vi "AODScanner_6_May_2014.vi"() -> ()   [LabVIEW 2012]
uses:
  AODAcq/AODAcq.lvclass
  <vilib>/rvi/interface/nirviReadWriteControl/nirviReadWriteControl.xnode
  FPGA_Control/AODRef.ctl
  <vilib>/rvi/interface/nirviMethod/nirviMethod.xnode
  <vilib>/rvi/errors/niLvFpgaMergeErrorWithErrorCode.vi
  Motion Stabilization/GlobalVars.vi
  <vilib>/DAQmx/write.llb/DAQmx Write (Analog DBL 1Chan 1Samp).vi
  <vilib>/DAQmx/read.llb/DAQmx Read (Analog Wfm 1Chan NSamp).vi
panel:
  out "Motion FIFO":refnum<queue>
  out "Motion ROIs":T1(array[cluster])
  out "Motion Plane Centers":i32[][](array[numeric])
  out "Number of Motion Planes":i32
  in  "Motion rate (Hz) 2":dbl=10.0
  out "error out 3":errorcluster
  out "Out Points":i32[][](array[numeric])
  out "Y-Z Motion Points":i32[][](array[numeric])
  out "X-Y Motion Points":i32[][](array[numeric])
  out "Points_um":dbl[][](array[numeric])
  out "Lens Magnification":i32=20
  in  "Matlab Server Shared Folder":string="c:\\temp"
  in  "Matlab Server IP Address":string="10.21.16.18"
  in  "External Magnification":dbl=1.3
  out "error out 2":errorcluster
  out "Objective Position":cluster{"X":dbl, "Y":dbl, "Z":dbl}
  out "Numeric":i32=299
  out "error out":errorcluster
  out "ROIs":T1(array[cluster])
  out "Histogram":dynamicdata(graph)
  out "Raw samples remaining":u32
  out "Temporal samples remaining":u32
  out "Motion samples remaining":u32
  out "Image samples remaining":u32
  out "Recording File":path
  out "Waveform Chart":waveform(dbl)(graph)
  out "Ephys":bool
  in  "TraceElements":u32=10000
  out "ScanProgress":dbl(slide) scale=0.0..1.0
  in  "Abort":bool
  out "Progress":dbl(slide) scale=0.0..1.0
  in  "SweepSettings":bool
  in  "stop":bool
  in  "Power":dbl(slide)=2.5 min=0.0 max=5.0 step=0.1 scale=0.0..2.5
  out "Scan":bool
  out "Volume":bool
  in  "Tab Control":enum32{"Setup", "Volume", "Traces", "Motion"}(tab)
  in  "Store Raw":bool
  in  "Disp Volume":bool=TRUE
  in  "Save Volume":bool
  in  "Ephys":bool
  in  "Motion rate (Hz)":dbl=10.0
  in  "Scan Settings (um)":T2={"XStart"=-100, "XEnd"=100, "XNum"=250, "YStart"=-100, "YEnd"=100, "YNum"=250, "ZStart"=-30, "ZEnd"=70, "ZNum"=60}
  in  "Objective":enum16{"20x Olympus"}(ring)
  in  "Scan Time (s)":dbl=300.0
  in  "Volume Reps":i32=1 min=1 max=10000
  in  "Volume":bool
  in  "Scan":bool
  in  "Motion Channel To Analyze":i32=2 min=1 max=2
  in  "Motion Analysis":bool
  in  "Per Cell Motion Analysis":bool
  in  "Sampling Structure":u16(ring) items=["Cube Vertices"]
  in  "Auto Motion Plane Params":T3={"XY Offset"=3, "Z Offset"=6, "Line Length"=12.0, "Box Size"=12.0, "Number of Planes Per Point"=3}
  in  "Mirror Ch1 Display":bool
  in  "ClearMotionCenters":bool
  in  "Point Centering":bool=TRUE
  in  "Recenter":bool caption="OK Button"
  out "Motion Points (Ch1)":u32
  out "Number selected":u32
  in  "Contrast":dbl(slide)=99.63636363636364 scale=98.0..100.0
  out "ImCh2":T4(plugin-control)
  out "ImCh1":T4(plugin-control)
  in  "Section":dbl min=0.0 max=59.0 step=1.0
  in  "Segment":bool
  out "Motion Increment":u32
  in  "Offset":dbl(slide)=0.010101010101010102 scale=0.0..1.0
  in  "ClearPoints":bool
  out "Total Motion Points":i32
  out "Motion Ch1":T4(plugin-control)
  out "Ephys":waveform(dbl)[](graph)
  out "Traces":waveform(dbl)[](graph)
  in  "Down Rate":i32=500
  in  "Spacing":dbl=100.0
  in  "Decimate":bool
  in  "Baseline Offset":dbl
  out "Motion Ch2":T4(plugin-control)
  out "Finished":bool
  out "Stopped":bool
  out "AODAcq out":refnum<class "AODAcq.lvclass">
  in  "Debug":bool
  in  "GridPoints":u16=10
  out "Scan Settings":T2
  out "VolData":i32[][](array[numeric])
  in  "VolumeElements":u32=10000
  in  "Points":i32[][](array[numeric])
  # "Off"
  # "On"
  # "On"
  # "Off"
  # "Off"
  # "On"
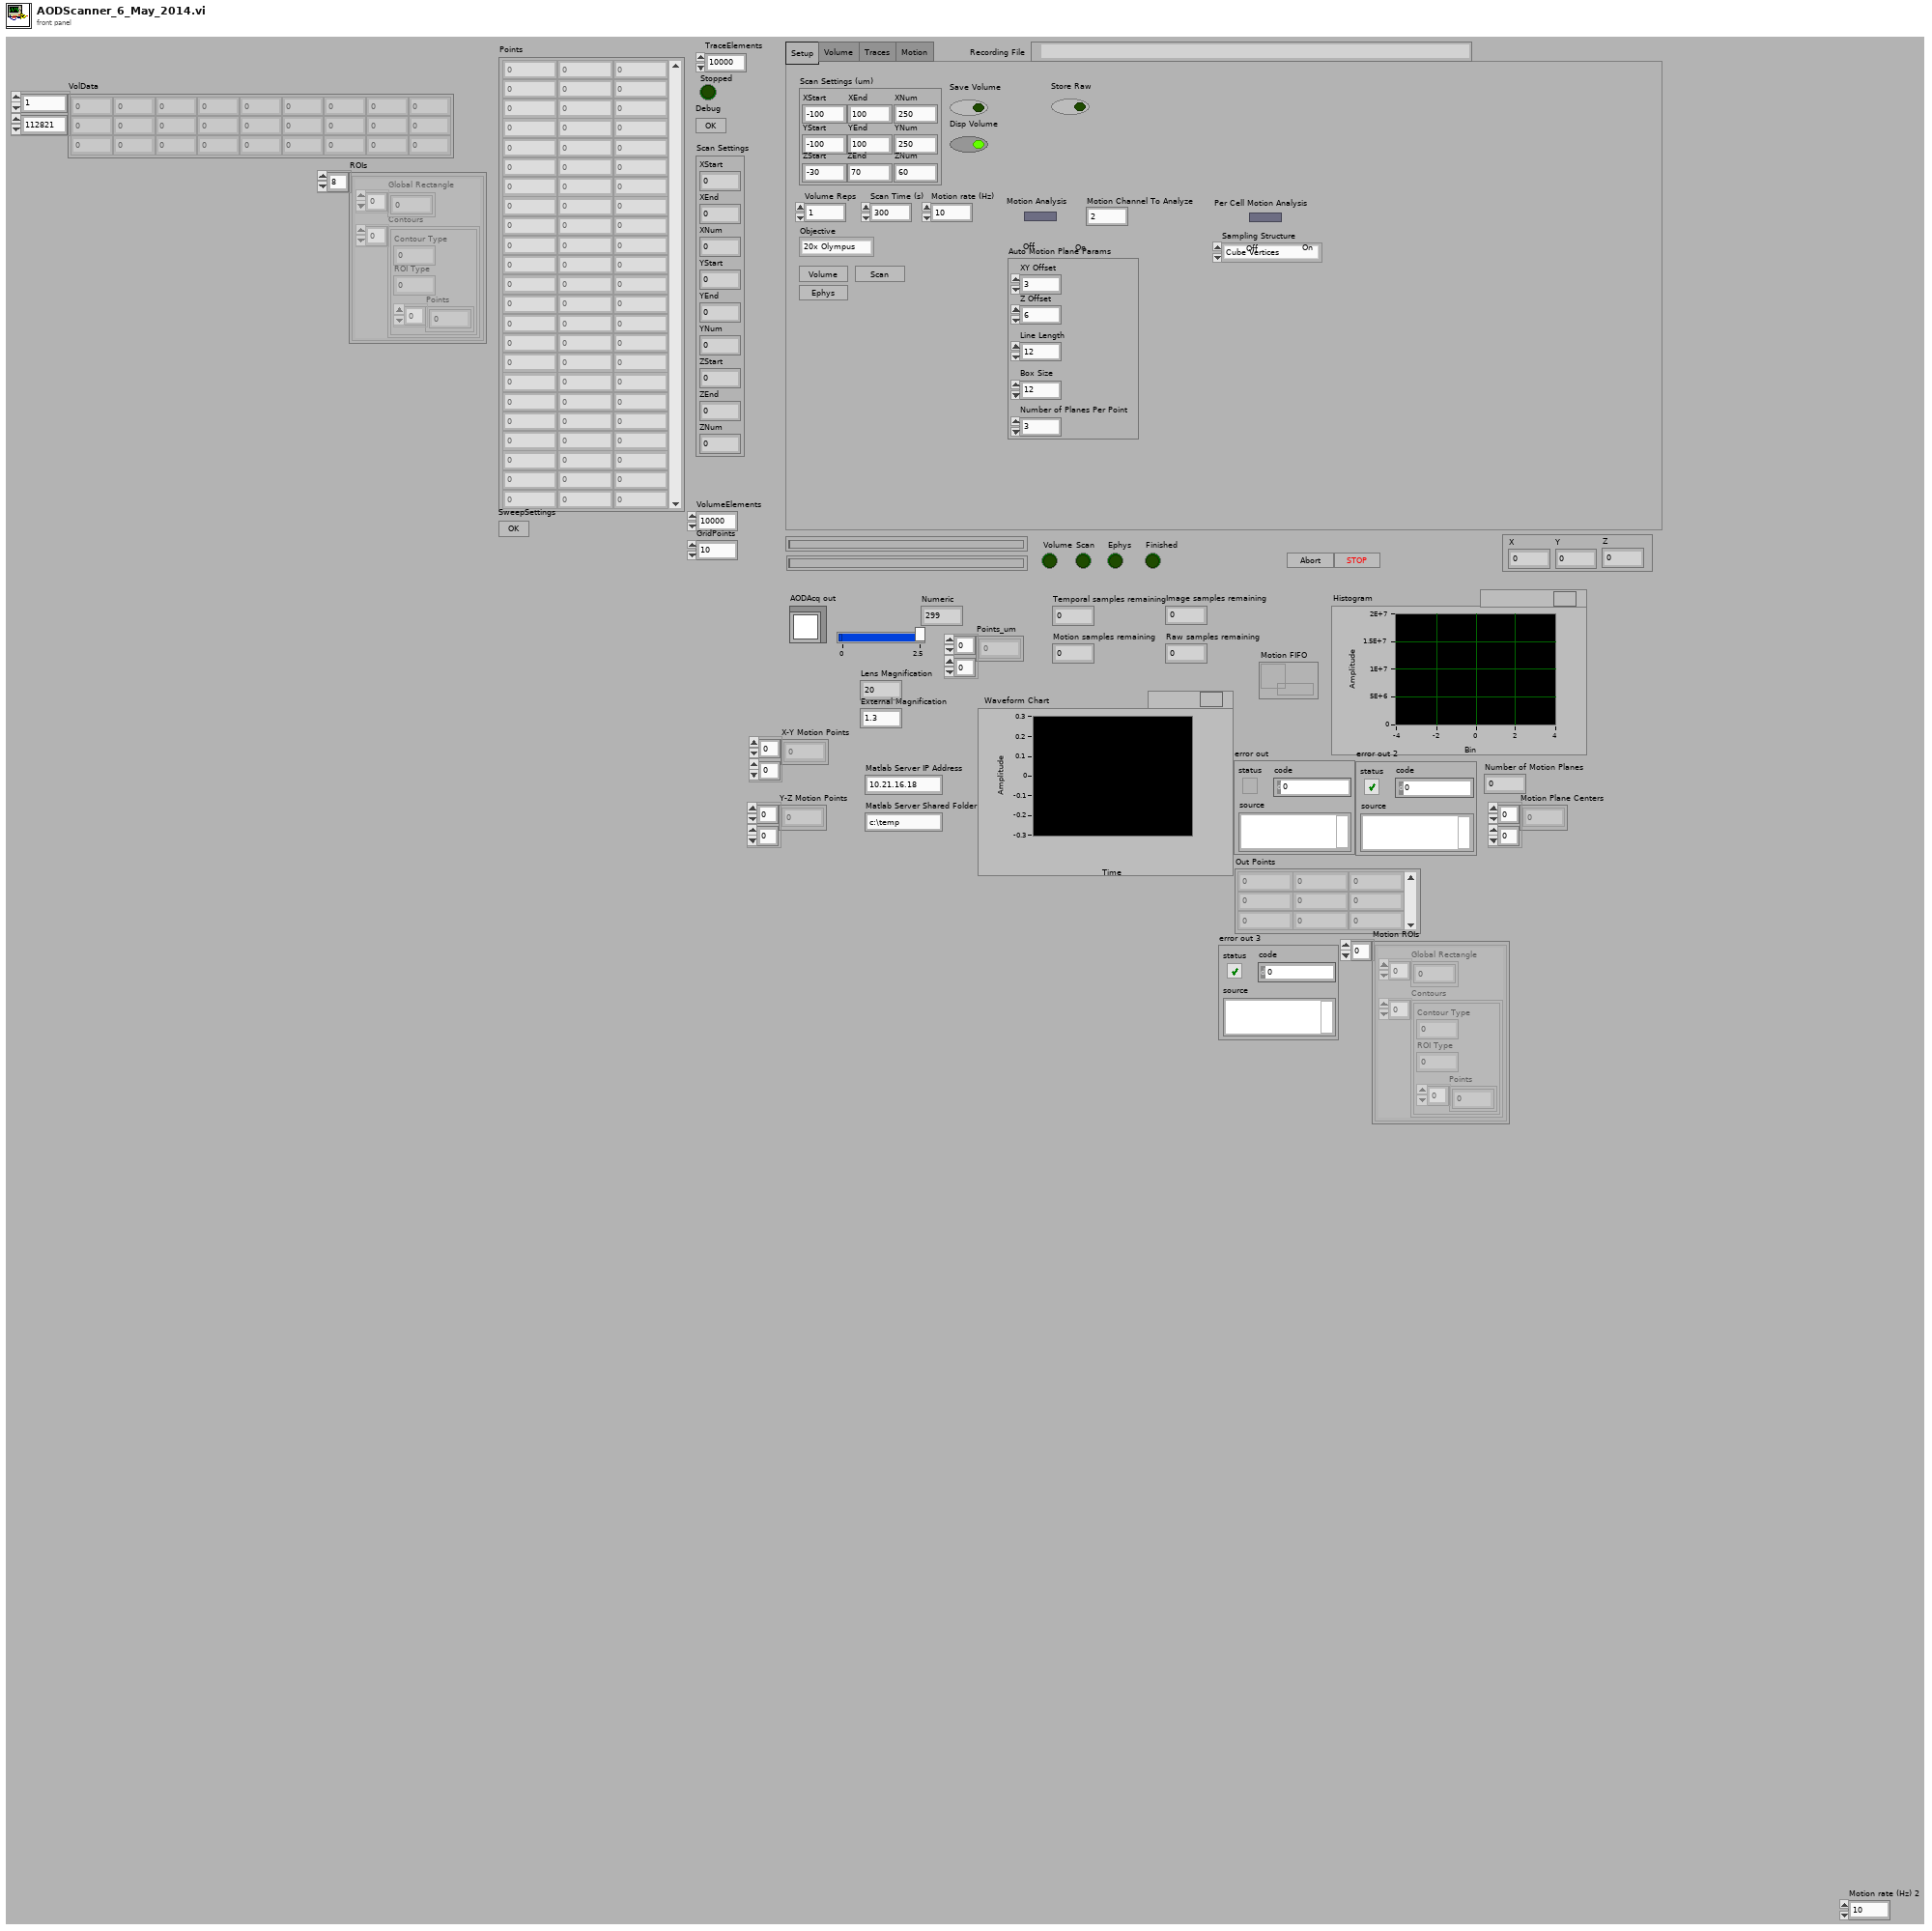
[diagram p1: front panel]
types:
  T1 = cluster{"Global Rectangle":i32[], "Contours":cluster{"Contour Type":u32, "ROI Type":u32, "Points":i32[]}[]}[]
  T2 = cluster{"XStart":i32, "XEnd":i32, "XNum":i32, "YStart":i32, "YEnd":i32, "YNum":i32, "ZStart":i32, "ZEnd":i32, "ZNum":i32}
  T3 = cluster{"XY Offset":i32, "Z Offset":i32, "Line Length":dbl, "Box Size":dbl, "Number of Planes Per Point":i32}
  T4 = typedef "IMAQ Image.ctl" = refnum<image>
  T5 = cluster{"gridsize":u16, "data":i32[][], "coordinates":i32[][], "settings":i32[], "settings_um":i32[], "needsreference":bool}
  T6 = typedef "Image Type" = u32
  T7 = cluster{"Global Rectangle":i32[], "Contours":cluster{"Contour Type":u32, "ROI Type":u32, "Points":i32[]}[]}
  T8 = cluster{"queue out":refnum<queue>, "queue out":refnum<queue>, "queue out":refnum<queue>}
  T9 = typedef "AODRef.ctl" = refnum<k20>
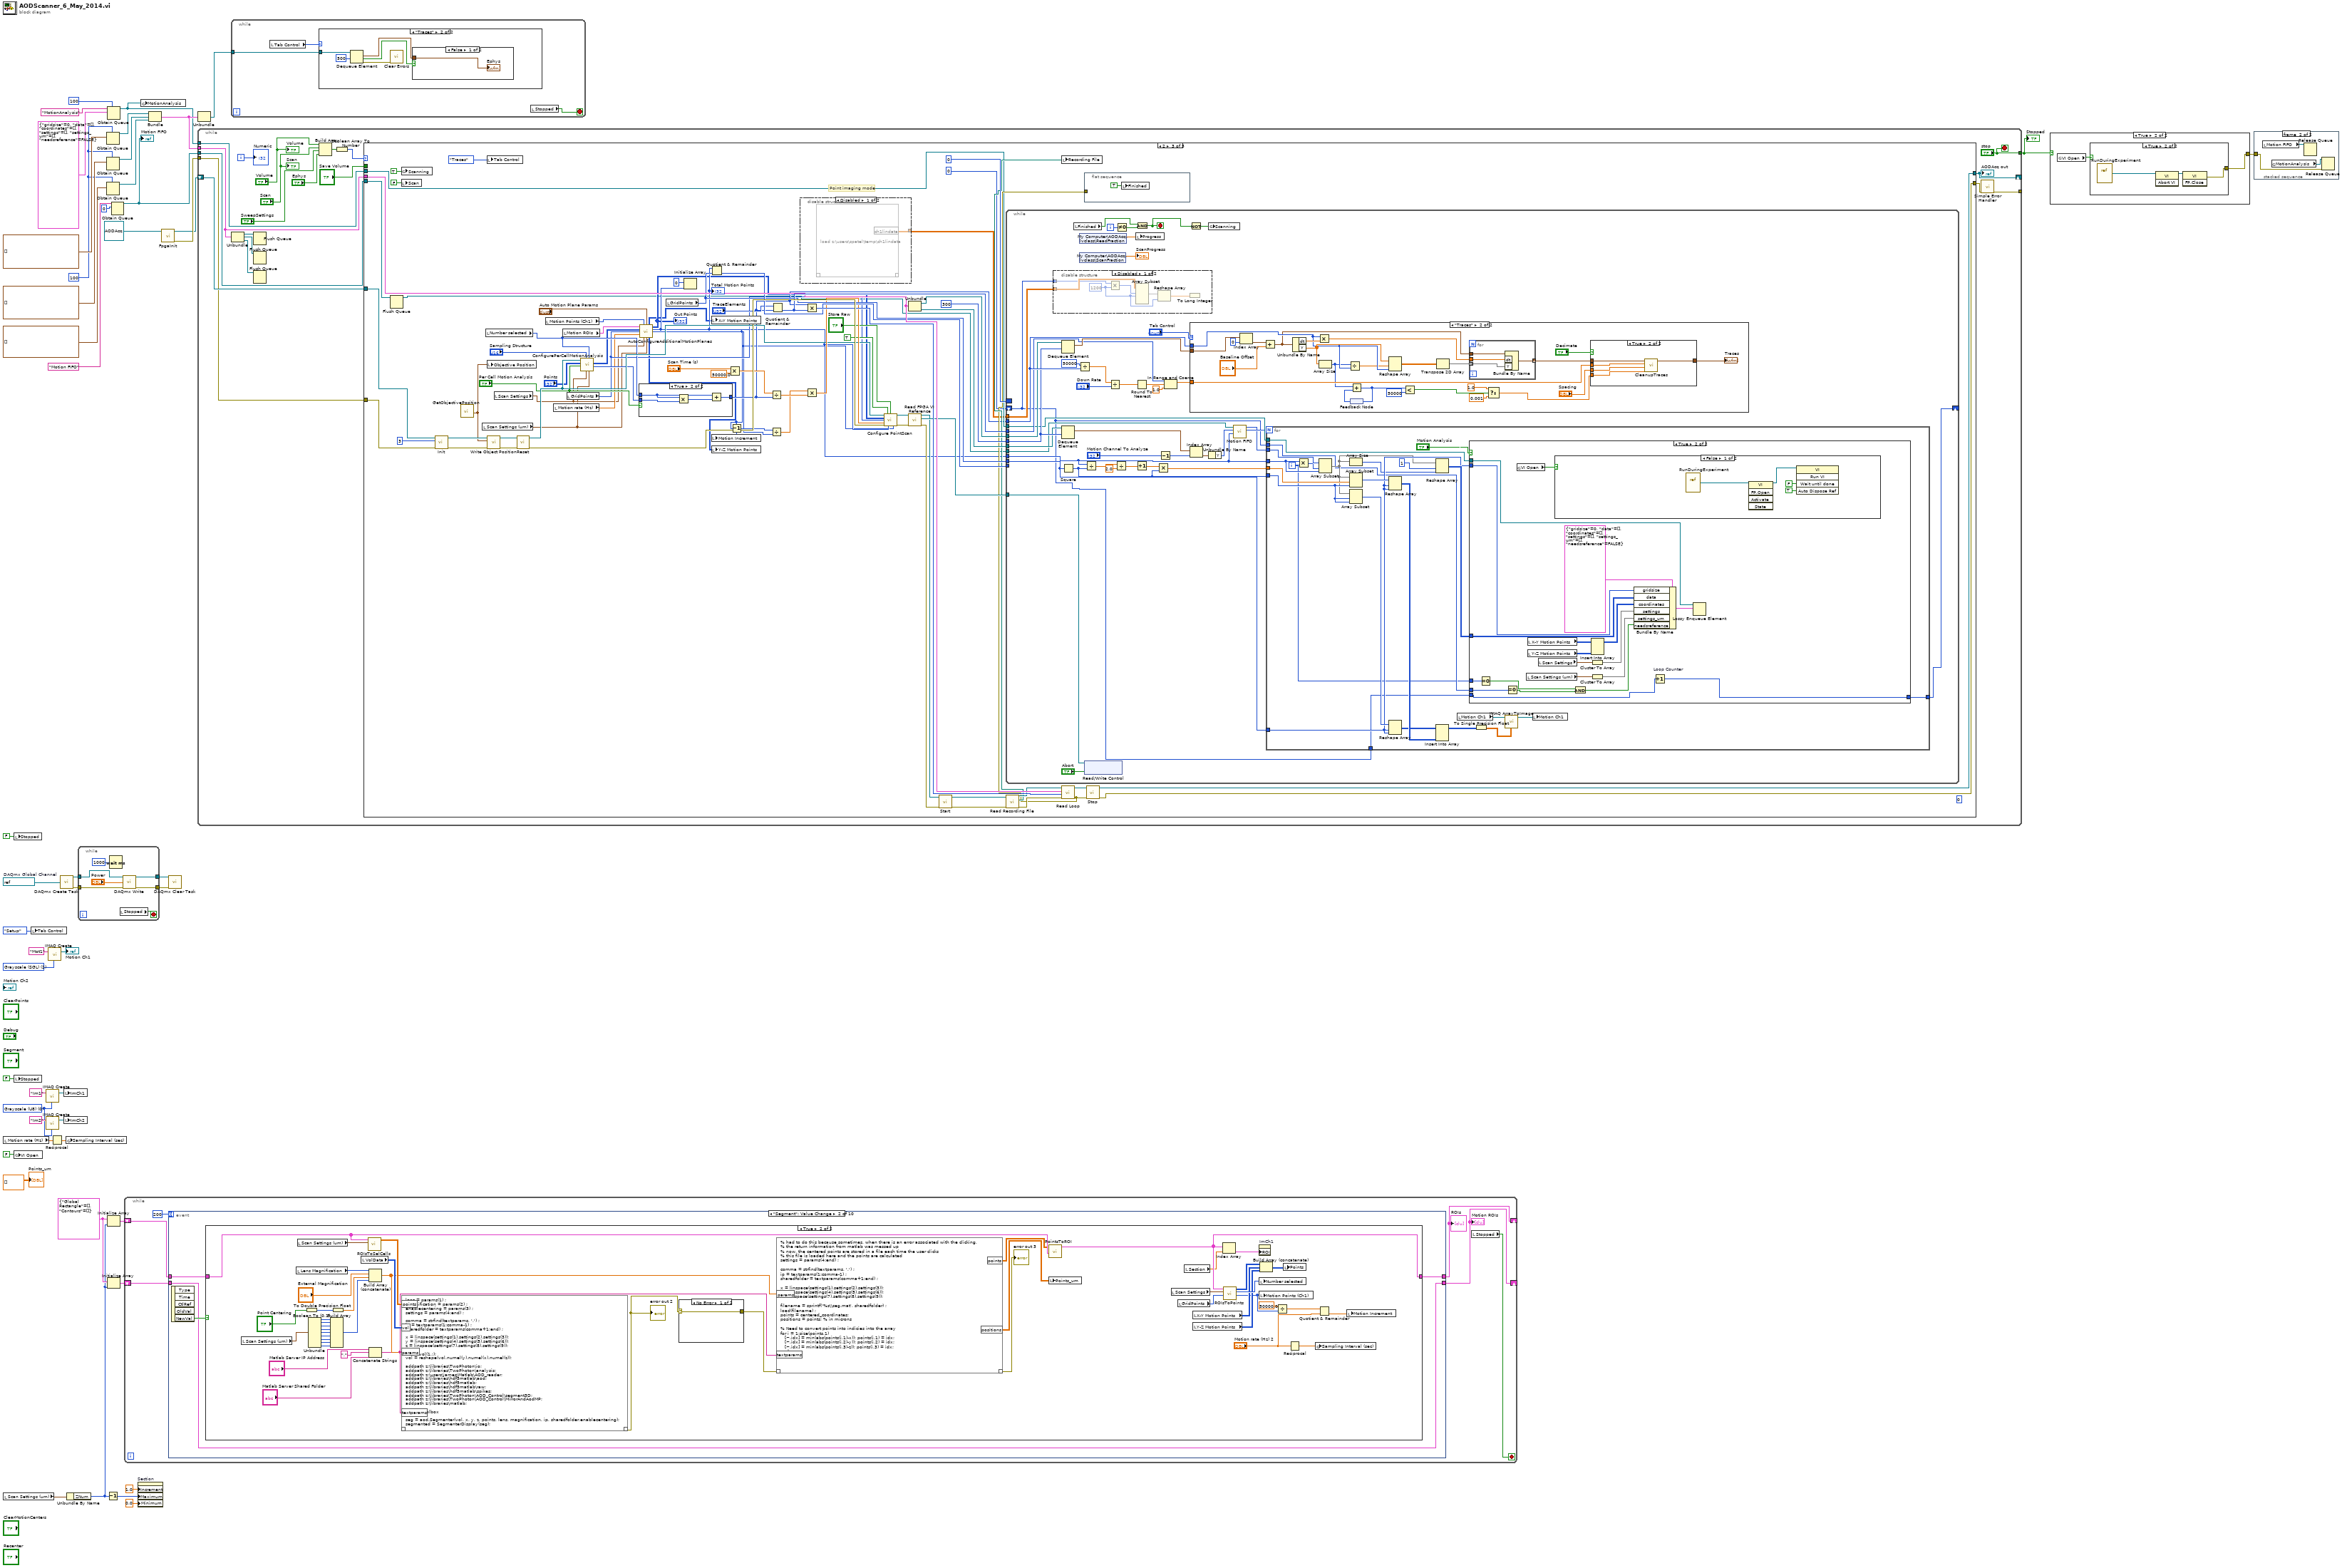
[diagram p0: block diagram]
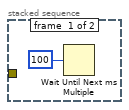
[diagram p2: hidden frame]
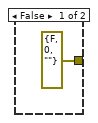
[diagram p3: hidden frame]
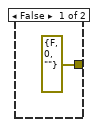
[diagram p4: hidden frame]
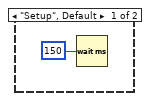
[diagram p5: hidden frame]
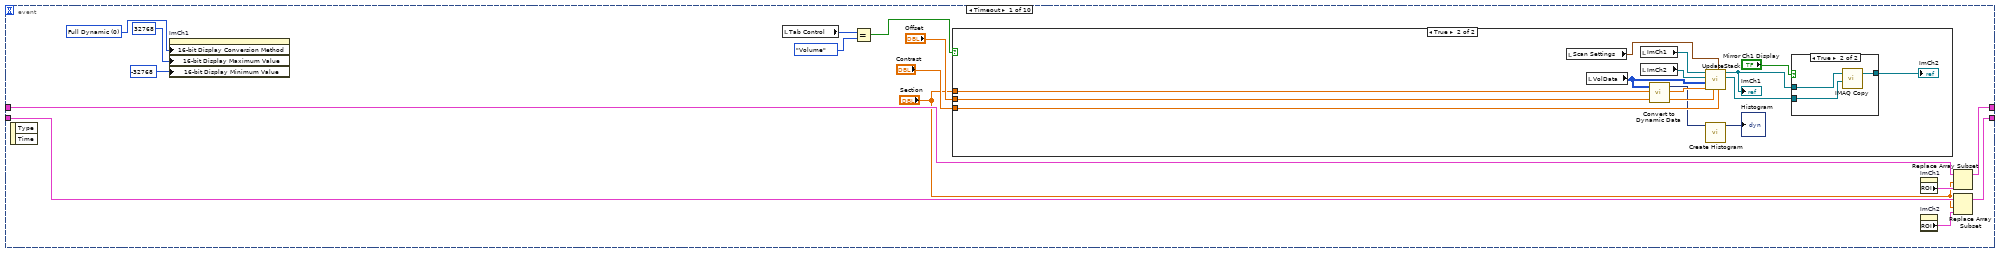
[diagram p7: hidden frame]
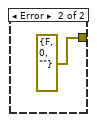
[diagram p11: hidden frame]
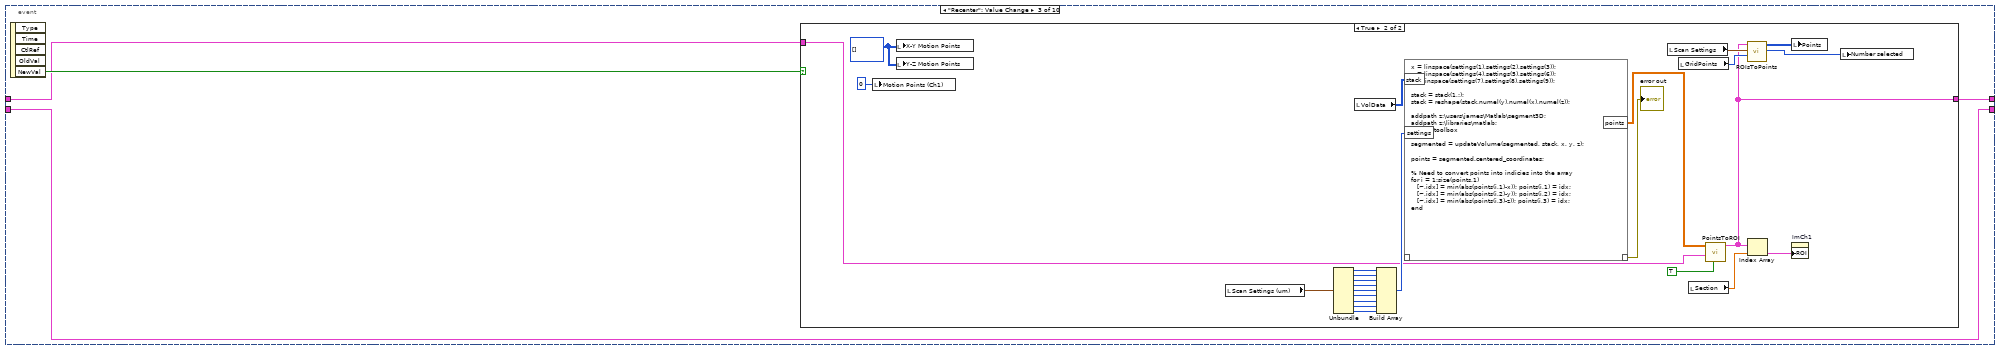
[diagram p12: hidden frame]
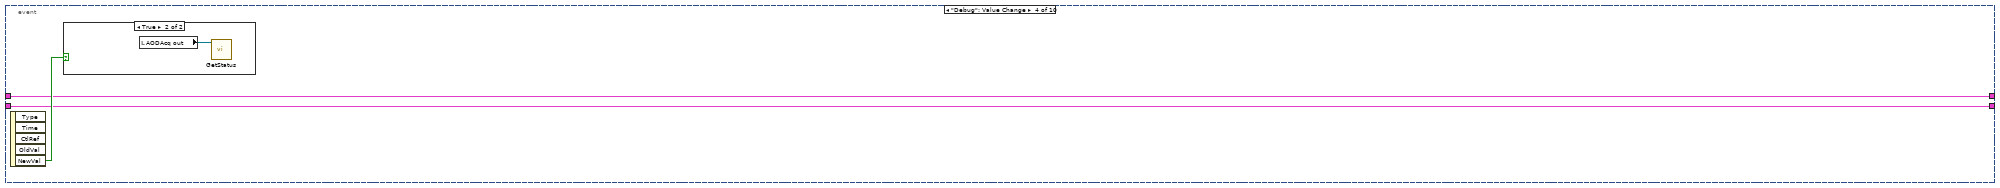
[diagram p14: hidden frame]
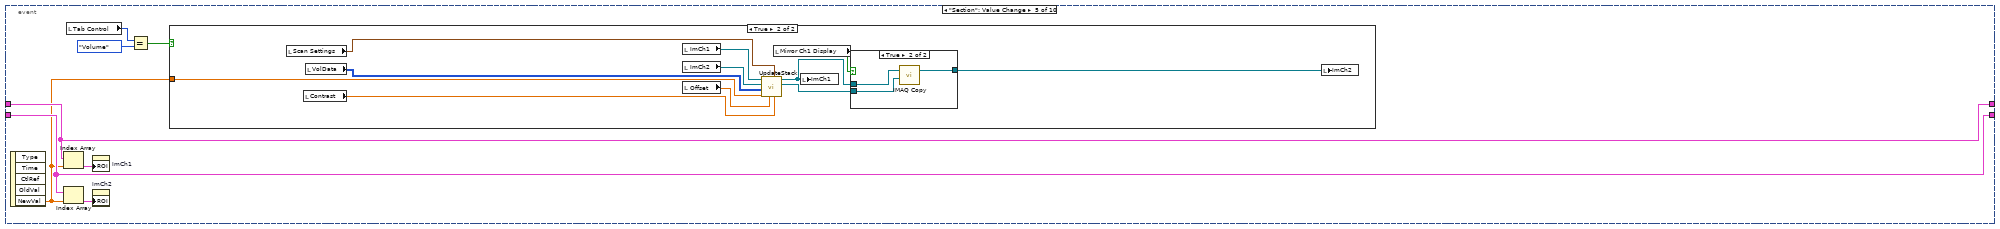
[diagram p16: hidden frame]
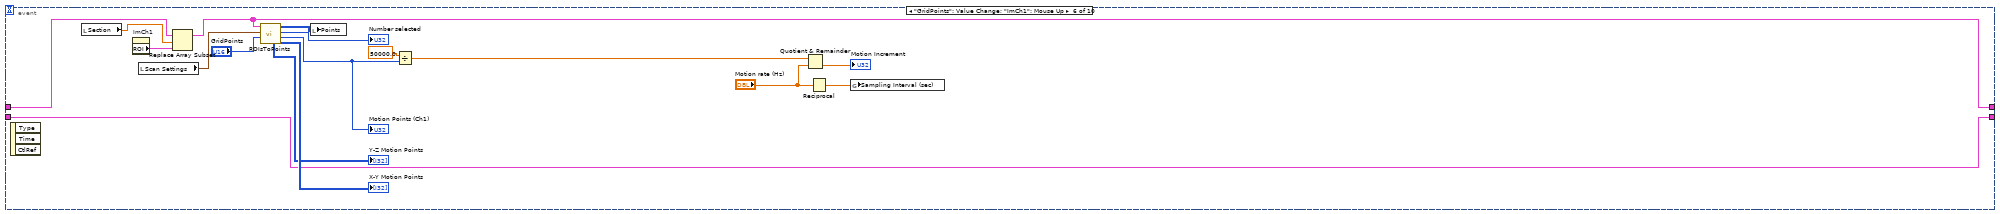
[diagram p19: hidden frame]
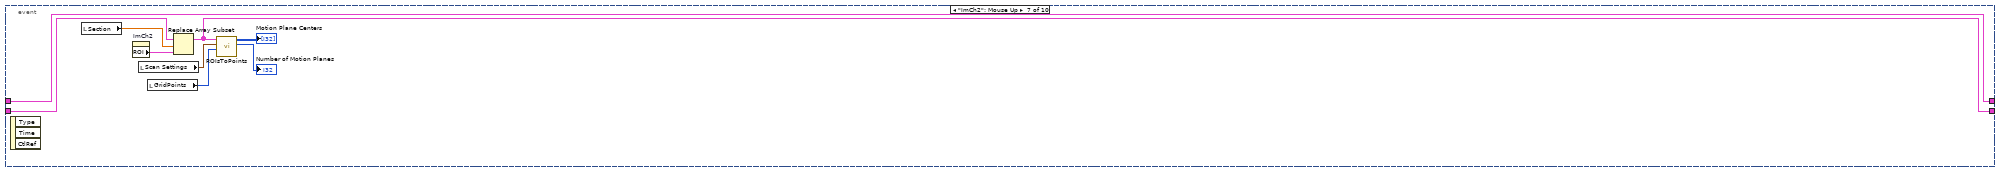
[diagram p20: hidden frame]
diagram:
  w18 = 100 ("max queue size (-1, unlimited)")
  w23 = T6 2 items=["Grayscale (U8)", "Grayscale (I16)", "Grayscale (SGL)", "Complex (CSG)", "RGB (U32)", "HSL (U32)", "RGB (U64)", "Grayscale (U16)"] ("Image Type")
  w34 = T6 0 items=["Grayscale (U8)", "Grayscale (I16)", "Grayscale (SGL)", "Complex (CSG)", "RGB (U32)", "HSL (U32)", "RGB (U64)", "Grayscale (U16)"] ("Image Type")
  w8 = T7 {"Global Rectangle"=[], "Contours"=[]} ("ROI")
  w44 = refnum<k21> "AOD Gain"  # DAQmx Global Channel
  n1 = local read "Motion rate (Hz)"() -> (w11:dbl)
  n2 = local read "Scan Settings (um)"() -> (w38:T2)
  n3 = local write "Stopped"(FALSE ("Stopped")) -> ()
  n4 = local write "Stopped"(FALSE ("Stopped")) -> ()
  n5 = global write "GlobalVars.vi" "VI Open"(FALSE ("VI Open")) -> ()
  n6 = local write "Tab Control"(enum32{"Setup", "Volume", "Traces", "Motion"}."Setup" ("Tab Control")) -> ()
  n7 = call "IMAQ Create"("Image Name"="Im1", "Image Type"=w34) -> ("New Image"=w46:T4)  [unwired: 3 in, 1 out]
  n8 = call "IMAQ Create"("Image Name"="Im2", "Image Type"=w34) -> ("New Image"=w45:T4)  [unwired: 3 in, 1 out]
  n9 = call "IMAQ Create"("Image Name"="Mot1", "Image Type"=w23) -> ("New Image"=→"Motion Ch1":T4)  [unwired: 3 in, 1 out]
  n10 = Reciprocal(x=w11) -> (1/x=w10:dbl)
  n11 = call <vilib>:"DAQmx Create Task.vi"("global virtual channels"=w44) -> ("task out"=w43:refnum<k21>, "error out"=w42:errorcluster)  [unwired: 4 in, 9 out]
  n12 = local write "ImCh1"(w46) -> ()
  n13 = local write "ImCh2"(w45) -> ()
  n14 = global write "GlobalVars.vi" "Sampling Interval (sec)"(w10) -> ()
  n15 = Unbundle By Name(w38) -> ("ZNum"=w7:i32)
  n16 = while {
    tunnel: w43 -> [w55]
    tunnel: w42 -> [w54]
    tunnel: [w53] -> w41
    tunnel: [w52] -> w40
    stop <- w51 stop-if-true
    n17 = Wait (ms)(milliseconds to wait=u32 1000) -> ()  [unwired: 1 out]
    n18 = local read "Stopped"() -> (w51:bool)
    n19 = call-poly <vilib>:"DAQmx Write.vi"("task/channels in"=w55, "data"="Power", "error in"=w54) -> ("task out"=w53:refnum<k21>, "error out"=w52:errorcluster)  [unwired: 10 in, 1 out]
  }
  n20 = Obtain Queue(max queue size (-1, unlimited)=w18, element data type=waveform(i32)[] []) -> (queue out=w29:refnum<queue>)  [unwired: 3 in, 2 out]
  n21 = Obtain Queue(max queue size (-1, unlimited)=w18, element data type=waveform(dbl)[] []) -> (queue out=w30:refnum<queue>)  [unwired: 3 in, 2 out]
  n22 = Obtain Queue(max queue size (-1, unlimited)=w18, element data type=waveform(i32)[] []) -> (queue out=w28:refnum<queue>)  [unwired: 3 in, 2 out]
  n23 = Decrement(x=w7) -> (x-1=w33:i32)
  n24 = Obtain Queue(max queue size (-1, unlimited)=100, name (unnamed)="MotionAnalysis", element data type=T5 {"gridsize"=0, "data"=[], "coordinates"=[], "settings"=[], "settings_um"=[], "needsreference"=FALSE}) -> (queue out=w1:refnum<queue>)  [unwired: 2 in, 2 out]
  n25 = Initialize Array(w8, w7) -> (w37:T1)
  n26 = Initialize Array(w8, w7) -> (w6:T1)
  n27 = Obtain Queue(name (unnamed)="Motion FIFO", element data type=0) -> (queue out=w3:refnum<queue>)  [unwired: 3 in, 2 out]
  "Motion FIFO" <- w3
  n28 = while {
    shift-right: [w61] -> _
    shift-left: w37 -> [w62]
    shift-right: [w58] -> _
    shift-left: w6 -> [w57]
    stop <- w59 stop-if-true
    n29 = event shown="[1] \"Segment\": Value Change" {
      selector: _ -> [_ _ _ _ _ _ _ _ _ _]
      dyn-events: _ -> [_ _ _ _ _ _ _ _ _ _]
      timeout: 200 -> [_ _ _ _ _ _ _ _ _ _]
      tunnel: w62 -> [w76 w97 w149 w179 w188 w221 w222 w235 w239 w251]
      tunnel: [w77 w96 w150 w179 w188 w218 w222 w234 w240 w251] -> w61
      tunnel: [w63 w95 w148 w178 w183 w205 w223 w231 w238 w252] -> w58
      tunnel: w57 -> [w66 w95 w148 w178 w183 w205 w228 w233 w238 w250]
      event Timeout {
        w71 = u32 0 items=["Full Dynamic", "Downshift", "Given Range", "90% Dynamic", "Given Percent Range"] ("16-bit Display Mapping:Conversion Method")
        n30 = event-data() -> ()  [unwired: 1 in, 2 out]
        n31 = property on="ImCh1" class="ImageControl"("16-bit Display Conversion Method"=w71, "16-bit Display Maximum Value"=32768 ("16-bit Display Mapping:Maximum Value"), "16-bit Display Minimum Value"=-32768 ("16-bit Display Mapping:Maximum Value")) -> ()  [unwired: 2 in, 2 out]
        n32 = local read "Tab Control"() -> (w74:enum32{"Setup", "Volume", "Traces", "Motion"})
        n33 = Equal?(x=w74, y=enum32{"Setup", "Volume", "Traces"}."Volume") -> (x = y?=w72:bool)
        n34 = case shown="True" w72 {
          tunnel: "Section" -> [_ w87]
          tunnel: "Offset" -> [_ w86]
          tunnel: "Contrast" -> [_ w85]
          frame False {
          }
          frame True {
            n35 = local read "Scan Settings"() -> (w88:T2)
            n36 = local read "VolData"() -> (w84:i32[][])
            n37 = local read "ImCh1"() -> (w90:T4)
            n38 = local read "ImCh2"() -> (w89:T4)
            n39 = call "Convert to Dynamic Data"("2D Array"=w84) -> ("Dynamic Data Type"=w83:dynamicdata)  [unwired: 3 in]
            n40 = call "UpdateStack.vi"("Contrast"=w85, "Scan Settings"=w88, "Offset"=w86, "Section"=w87, "ImData"=w84, "Im2 2"=w89, "Im1 In"=w90) -> ("Im2 Out"=w78:T4, "Im1 Out"=w80:T4)  [unwired: 3 in]
            "ImCh1" <- w80
            n41 = call "Create Histogram"("Signal"=w83) -> ("Histogram"=→"Histogram":dynamicdata)  [unwired: 9 in, 1 out]
            n42 = case shown="True" "Mirror Ch1 Display" {
              tunnel: w80 -> [_ w93]
              tunnel: [w91 w92] -> w79
              tunnel: w78 -> [w91 w94]
              frame False {
              }
              frame True {
                n43 = call "IMAQ Copy"("Image Dst"=w94, "Image Src"=w93) -> ("Image Dst Out"=w92:T4)  [unwired: 4 in, 1 out]
              }
            }
            "ImCh2" <- w79
          }
        }
        n44 = property on="ImCh1" class="ImageControl"() -> ("ROI"=w75:T7)  [unwired: 2 in, 2 out]
        n45 = property on="ImCh2" class="ImageControl"() -> ("ROI"=w65:T7)  [unwired: 2 in, 2 out]
        n46 = Replace Array Subset(array=w76, new element=w75, index="Section") -> (w77:T1)
        n47 = Replace Array Subset(array=w66, new element=w65, index="Section") -> (w63:T1)
      }
      event "Segment": Value Change {
        n48 = event-data() -> ("NewVal"=w98:bool)  [unwired: 1 in, 4 out]
        n49 = case shown="True" w98 {
          tunnel: w97 -> [w99 w123]
          tunnel: [w99 w131] -> w96
          frame False {
          }
          frame True {
            n50 = local read "Scan Settings (um)"() -> (w145:T2)
            n51 = local read "Lens Magnification"() -> (w119:i32)
            n52 = local read "Scan Settings (um)"() -> (w121:T2)
            n53 = Boolean To (0,1)(Boolean="Point Centering") -> (0, 1=w124:i16)
            n54 = Unbundle(w145) -> ("XStart"=w144:i32, "XEnd"=w143:i32, "XNum"=w142:i32, "YStart"=w141:i32, "YEnd"=w140:i32, "YNum"=w139:i32, "ZStart"=w138:i32, "ZEnd"=w137:i32, "ZNum"=w136:i32)
            n55 = Build Array(w144, w143, w142, w141, w140, w139, w138, w137, w136) -> (w113:i32[])
            n56 = To Double Precision Float(number=w124) -> (double precision float=w117:dbl)
            n57 = local read "VolData"() -> (w135:i32[][])
            n58 = call "ROIsToSelCells.vi"("Scan Settings"=w121, "ROI"=w123) -> ("Points_um"=w120:dbl[][])  [unwired: 8 in, 1 out]
            n59 = Concatenate Strings("Matlab Server IP Address", "," ("string"), "Matlab Server Shared Folder") -> (w109:string)
            n60 = Build Array (concatenate)(w119, "External Magnification", w117, w113) -> (w110:dbl[])
            n61 = script code="lens = params(1) ;\nmagnification = params(2) ;\nenablecentering = params(3) ;\nsettings = params(4:end) ;\n\ncomma = strfind(textparams, ',') ;\nip = textparams(1:comma-1) ;\nsharedfolder = textparams(comma+1:end) ;\n\nx = linspace(settings(1),settings(2),settings(3));\ny = linspace(settings(4),settings(5),settings(6));\nz = linspace(settings(7),settings(8),settings(9));\n\nvol = vol(1,:);\nvol = reshape(vol,numel(y),numel(x),numel(z));\n\naddpath z:\\libraries\\TwoPhoton\\io;\naddpath z:\\libraries\\TwoPhoton\\analysis;\naddpath z:\\users\\james\\Matlab\\AOD_reader;\naddpath z:\\libraries\\hdf5matlab\\aod;\naddpath z:\\libraries\\hdf5matlab;\naddpath z:\\libraries\\hdf5matlab\\raw;\naddpath z:\\libraries\\hdf5matlab\\spikes;\naddpath z:\\libraries\\TwoPhoton\\AOD_Control\\segment3D;\naddpath z:\\libraries\\TwoPhoton\\AOD_Control\\MirrorAndAodMP;\naddpath z:\\libraries\\matlab;\n\nrehash toolbox\n\nseg = aod.Segmenter(vol, x, y, z, points, lens, magnification, ip, sharedfolder,enablecentering);\nsegmented = SegmenterDisplay(seg);"("vol"=w135, "params"=w110, "textparams"=w109, "points"=w120) -> ("??"=w107:errorcluster)  [unwired: 1 in]
            "error out 2" <- w107
            n62 = case shown="No Error" w107 {
              selector: w107 -> [w146 _]
              tunnel: [w146 errorcluster {"status"=FALSE, "code"=0, "source"=""} ("error IO")] -> w106
              frame No Error {
              }
              frame Error {
              }
            }
            n63 = script code="% had to do this because sometimes, when there is an error associated with the clicking,\n% the return information from matlab was messed up\n% now, the centered points are stored in a file each time the user clicks\n% this file is loaded here and the points are calculated\nsettings = params(4:end) ;\n\ncomma = strfind(textparams, ',') ;\nip = textparams(1:comma-1) ;\nsharedfolder = textparams(comma+1:end) ;\n\nx = linspace(settings(1),settings(2),settings(3));\ny = linspace(settings(4),settings(5),settings(6));\nz = linspace(settings(7),settings(8),settings(9));\n\nfilename = sprintf('%s\\\\seg.mat', sharedfolder) ;\nload(filename) ;\npoints = centered_coordinates;\npositions = points; % in microns\n\n% Need to convert points into indicies into the array\nfor i = 1:size(points,1)\n   [~,idx] = min(abs(points(i,1)-x)); points(i,1) = idx;\n   [~,idx] = min(abs(points(i,2)-y)); points(i,2) = idx;\n   [~,idx] = min(abs(points(i,3)-z)); points(i,3) = idx;\nend"("??"=w106, "params"=w110, "textparams"=w109) -> ("??"=→"error out 3":errorcluster, "points"=w112:dbl[][], "positions"=w111:dbl[][])
            n64 = call "PointsToROI.vi"("Old ROIs"=w123, "Points"=w112) -> ("ROIs"=w131:T1)  [unwired: 9 in]
            n65 = local write "Points_um"(w111) -> ()
            n66 = local read "Scan Settings"() -> (w133:T2)
            n67 = local read "GridPoints"() -> (w122:u16)
            n68 = local read "Section"() -> (w130:dbl)
            n69 = local read "X-Y Motion Points"() -> (w127:i32[][])
            n70 = local read "Y-Z Motion Points"() -> (w126:i32[][])
            n71 = Index Array(array=w131, index=w130) -> (element=w132:T7)
            n72 = call "ROIsToPoints.vi"("GridPoints"=w122, "Scan Settings"=w133, "ROI"=w131) -> ("Number of motion points"=w100:i32, "Number of points"=w134:i32, "Points"=w129:i32[][])  [unwired: 4 in, 2 out]
            n73 = property on="ImCh1" class="ImageControl"("ROI"=w132) -> ()  [unwired: 2 in, 2 out]
            n74 = local write "Number selected"(w134) -> ()
            n75 = local write "Motion Points (Ch1)"(w100) -> ()
            n76 = Build Array (concatenate)(w129, w127, w126) -> (w128:i32[][])
            n77 = Divide(x=50000.0, y=w100) -> (x/y=w102:dbl)
            n78 = local write "Points"(w128) -> ()
            n79 = Reciprocal(x="Motion rate (Hz) 2") -> (1/x=w103:dbl)
            n80 = global write "GlobalVars.vi" "Sampling Interval (sec)"(w103) -> ()
            n81 = Quotient & Remainder(x=w102, y="Motion rate (Hz) 2") -> (floor(x/y)=w101:dbl)  [unwired: 1 out]
            n82 = local write "Motion Increment"(w101) -> ()
          }
        }
      }
      event "Recenter": Value Change {
        n83 = event-data() -> ("NewVal"=w151:bool)  [unwired: 1 in, 4 out]
        n84 = case shown="True" w151 {
          tunnel: [w152 w157] -> w150
          tunnel: w149 -> [w152 w160]
          frame False {
          }
          frame True {
            w155 = i32[][] [] ("Points")
            n85 = local write "Motion Points (Ch1)"(u32 0 ("Number of Motion Points")) -> ()
            n86 = local write "X-Y Motion Points"(w155) -> ()
            n87 = local write "Y-Z Motion Points"(w155) -> ()
            n88 = local read "Scan Settings (um)"() -> (w163:T2)
            n89 = Unbundle(w163) -> ("XStart"=w177:i32, "XEnd"=w176:i32, "XNum"=w175:i32, "YStart"=w174:i32, "YEnd"=w173:i32, "YNum"=w172:i32, "ZStart"=w171:i32, "ZEnd"=w170:i32, "ZNum"=w169:i32)
            n90 = local read "VolData"() -> (w167:i32[][])
            n91 = Build Array(w177, w176, w175, w174, w173, w172, w171, w170, w169) -> (w168:i32[])
            n92 = script code="x = linspace(settings(1),settings(2),settings(3));\ny = linspace(settings(4),settings(5),settings(6));\nz = linspace(settings(7),settings(8),settings(9));\n\nstack = stack(1,:);\nstack = reshape(stack,numel(y),numel(x),numel(z));\n\naddpath z:\\users\\james\\Matlab\\segment3D;\naddpath z:\\libraries\\matlab;\nrehash toolbox\n\nsegmented = updateVolume(segmented, stack, x, y, z);\n\npoints = segmented.centered_coordinates;\n\n% Need to convert points into indicies into the array\nfor i = 1:size(points,1)\n   [~,idx] = min(abs(points(i,1)-x)); points(i,1) = idx;\n   [~,idx] = min(abs(points(i,2)-y)); points(i,2) = idx;\n   [~,idx] = min(abs(points(i,3)-z)); points(i,3) = idx;\nend"("stack"=w167, "settings"=w168) -> ("??"=→"error out":errorcluster, "points"=w166:dbl[][])  [unwired: 1 in]
            n93 = local read "Scan Settings"() -> (w162:T2)
            n94 = local read "GridPoints"() -> (w164:u16)
            n95 = local read "Section"() -> (w158:dbl)
            n96 = call "PointsToROI.vi"("Clear Motion Planes"=TRUE, "Old ROIs"=w160, "Points"=w166) -> ("ROIs"=w157:T1)  [unwired: 8 in]
            n97 = call "ROIsToPoints.vi"("GridPoints"=w164, "Scan Settings"=w162, "ROI"=w157) -> ("Number of points"=w165:i32, "Points"=w156:i32[][])  [unwired: 4 in, 3 out]
            n98 = Index Array(array=w157, index=w158) -> (element=w159:T7)
            n99 = local write "Points"(w156) -> ()
            n100 = property on="ImCh1" class="ImageControl"("ROI"=w159) -> ()  [unwired: 2 in, 2 out]
            n101 = local write "Number selected"(w165) -> ()
          }
        }
      }
      event "Debug": Value Change {
        n102 = event-data() -> ("NewVal"=w180:bool)  [unwired: 1 in, 4 out]
        n103 = case shown="True" w180 {
          frame False {
          }
          frame True {
            n104 = local read "AODAcq out"() -> (w181:refnum<class "AODAcq.lvclass">)
            n105 = call-dynamic "GetStatus.vi"("AODAcq in"=w181) -> ()  [unwired: 8 in, 3 out]
          }
        }
      }
      event "Section": Value Change {
        n106 = event-data() -> ("NewVal"=w182:dbl)  [unwired: 1 in, 4 out]
        n107 = Index Array(array=w188, index=w182) -> (element=w189:T7)
        n108 = Index Array(array=w183, index=w182) -> (element=w184:T7)
        n109 = local read "Tab Control"() -> (w187:enum32{"Setup", "Volume", "Traces", "Motion"})
        n110 = property on="ImCh1" class="ImageControl"("ROI"=w189) -> ()  [unwired: 2 in, 2 out]
        n111 = property on="ImCh2" class="ImageControl"("ROI"=w184) -> ()  [unwired: 2 in, 2 out]
        n112 = Equal?(x=w187, y=enum32{"Setup", "Volume", "Traces"}."Volume") -> (x = y?=w185:bool)
        n113 = case shown="True" w185 {
          tunnel: w182 -> [_ w197]
          frame False {
          }
          frame True {
            n114 = local read "Scan Settings"() -> (w196:T2)
            n115 = local read "Contrast"() -> (w194:dbl)
            n116 = local read "VolData"() -> (w200:i32[][])
            n117 = local read "ImCh1"() -> (w198:T4)
            n118 = local read "ImCh2"() -> (w199:T4)
            n119 = local read "Offset"() -> (w195:dbl)
            n120 = call "UpdateStack.vi"("Contrast"=w194, "Scan Settings"=w196, "Offset"=w195, "Section"=w197, "ImData"=w200, "Im2 2"=w199, "Im1 In"=w198) -> ("Im2 Out"=w192:T4, "Im1 Out"=w193:T4)  [unwired: 3 in]
            n121 = local read "Mirror Ch1 Display"() -> (w190:bool)
            n122 = local write "ImCh1"(w193) -> ()
            n123 = case shown="True" w190 {
              tunnel: w193 -> [_ w203]
              tunnel: [w201 w202] -> w191
              tunnel: w192 -> [w201 w204]
              frame False {
              }
              frame True {
                n124 = call "IMAQ Copy"("Image Dst"=w204, "Image Src"=w203) -> ("Image Dst Out"=w202:T4)  [unwired: 4 in, 1 out]
              }
            }
            n125 = local write "ImCh2"(w191) -> ()
          }
        }
      }
      event "GridPoints": Value Change; "ImCh1": Mouse Up {
        n126 = event-data() -> ()  [unwired: 1 in, 3 out]
        n127 = local read "Section"() -> (w219:dbl)
        n128 = property on="ImCh1" class="ImageControl"() -> ("ROI"=w220:T7)  [unwired: 2 in, 2 out]
        n129 = local read "Scan Settings"() -> (w217:T2)
        n130 = Replace Array Subset(array=w221, new element=w220, index=w219) -> (w218:T1)
        n131 = call "ROIsToPoints.vi"("GridPoints"="GridPoints", "Scan Settings"=w217, "ROI"=w218) -> ("X-Y Motion Points"=→"X-Y Motion Points":i32[][], "Number of motion points"=w212:i32, "Number of points"=→"Number selected":i32, "Points"=w215:i32[][], "Y-Z Motion Points"=→"Y-Z Motion Points":i32[][])  [unwired: 4 in]
        "Motion Points (Ch1)" <- w212
        n132 = local write "Points"(w215) -> ()
        n133 = Divide(x=50000.0, y=w212) -> (x/y=w211:dbl)
        n134 = Quotient & Remainder(x=w211, y="Motion rate (Hz)") -> (floor(x/y)=→"Motion Increment":dbl)  [unwired: 1 out]
        n135 = Reciprocal(x="Motion rate (Hz)") -> (1/x=w208:dbl)
        n136 = global write "GlobalVars.vi" "Sampling Interval (sec)"(w208) -> ()
      }
      event "ImCh2": Mouse Up {
        n137 = event-data() -> ()  [unwired: 1 in, 3 out]
        n138 = local read "Section"() -> (w229:dbl)
        n139 = property on="ImCh2" class="ImageControl"() -> ("ROI"=w230:T7)  [unwired: 2 in, 2 out]
        n140 = local read "Scan Settings"() -> (w227:T2)
        n141 = local read "GridPoints"() -> (w226:u16)
        n142 = Replace Array Subset(array=w228, new element=w230, index=w229) -> (w223:T1)
        n143 = call "ROIsToPoints.vi"("GridPoints"=w226, "Scan Settings"=w227, "ROI"=w223) -> ("Number of points"=→"Number of Motion Planes":i32, "Points"=→"Motion Plane Centers":i32[][])  [unwired: 4 in, 3 out]
      }
      event "Scan Settings (um).ZNum": Value Change {
        n144 = event-data() -> ("NewVal"=w232:i32)  [unwired: 1 in, 4 out]
        n145 = Decrement(x=w232) -> (x-1=w236:i32)
        n146 = property on="Section" class="DigNum (strict)"("Maximum"=w236, "Minimum"=0.0 ("Data Entry Limits:Minimum")) -> ()  [unwired: 2 in, 2 out]
        n147 = Reshape Array(w235, w232) -> (w234:T1)
        n148 = Reshape Array(w233, w232) -> (w231:T1)
      }
      event "ClearPoints": Value Change {
        n149 = event-data() -> ("NewVal"=w241:bool)  [unwired: 1 in, 4 out]
        n150 = case shown="True" w241 {
          tunnel: [w242 w249] -> w240
          tunnel: w239 -> [w242 _]
          frame False {
          }
          frame True {
            w243 = u32 0 ("Number of Motion Points")
            w244 = i32[][] [] ("Points")
            w248 = T7 {"Global Rectangle"=[], "Contours"=[]} ("ROI")
            n151 = local write "Points_um"(dbl[][] [] ("Points_um")) -> ()
            n152 = local write "Number selected"(w243) -> ()
            n153 = local write "Motion Points (Ch1)"(w243) -> ()
            n154 = local write "Points"(w244) -> ()
            n155 = local read "Scan Settings"() -> (w247:T2)
            n156 = local write "Y-Z Motion Points"(w244) -> ()
            n157 = local write "X-Y Motion Points"(w244) -> ()
            n158 = property on="ImCh1" class="ImageControl"("ROI"=w248) -> ()  [unwired: 2 in, 2 out]
            n159 = Unbundle By Name(w247) -> ("ZNum"=w246:i32)
            n160 = Initialize Array(w248, w246) -> (w249:T1)
          }
        }
      }
      event "ClearMotionCenters": Value Change {
        n161 = event-data() -> ("NewVal"=w253:bool)  [unwired: 1 in, 4 out]
        n162 = case shown="True" w253 {
          tunnel: [w254 w255] -> w252
          tunnel: w250 -> [w254 _]
          frame False {
          }
          frame True {
            w256 = T7 {"Global Rectangle"=[], "Contours"=[]} ("ROI")
            n163 = local read "Scan Settings"() -> (w258:T2)
            n164 = property on="ImCh2" class="ImageControl"("ROI"=w256) -> ()  [unwired: 2 in, 2 out]
            n165 = Unbundle By Name(w258) -> ("ZNum"=w257:i32)
            n166 = Initialize Array(w256, w257) -> (w255:T1)
          }
        }
      }
    }
    "ROIs" <- w61
    "Motion ROIs" <- w58
    n167 = local read "Stopped"() -> (w59:bool)
  }
  n168 = property on="Section" class="DigNum (strict)"("Increment"=1.0 ("Data Entry Limits:Increment"), "Maximum"=w33, "Minimum"=0.0 ("Data Entry Limits:Minimum")) -> ()  [unwired: 2 in, 2 out]
  n169 = global write "GlobalVars.vi" "MotionAnalysis"(w1) -> ()
  n170 = Bundle("queue out"=w29, "queue out"=w30, "queue out"=w28) -> (w27:T8)  [unwired: 1 in]
  n171 = call-dynamic "FpgaInit.vi"("AODAcq in"=refnum<class "AODAcq.lvclass"> refnum ("AODAcq.lvclass")) -> ("error out"=w21:errorcluster, "AODAcq out"=w20:refnum<class "AODAcq.lvclass">)  [unwired: 9 in]
  n172 = call <vilib>:"DAQmx Clear Task.vi"("task in"=w41, "error in"=w40) -> ()  [unwired: 13 in, 1 out]
  n173 = Unbundle(w27) -> ("queue out"=w26:refnum<queue>)  [unwired: 2 out]
  n174 = while {
    shift-right: [w272] -> _
    shift-left: w20 -> [w278]
    tunnel: w27 -> [w262]
    tunnel: w21 -> [w277]
    tunnel: [w270] -> _
    tunnel: ["stop"] -> w12
    tunnel: w1 -> [w264]
    tunnel: w3 -> [w263]
    i -> [w265]
    stop <- "stop" stop-if-true
    n175 = Unbundle(w262) -> ("queue out"=w261:refnum<queue>, "queue out"=w260:refnum<queue>, "queue out"=w259:refnum<queue>)
    n176 = Flush Queue(queue=w261) -> ()  [unwired: 1 in, 3 out]
    n177 = Flush Queue(queue=w260) -> ()  [unwired: 1 in, 3 out]
    n178 = Flush Queue(queue=w259) -> ()  [unwired: 1 in, 3 out]
    n179 = Build Array("Volume", "Scan", "SweepSettings", "Ephys") -> (w274:bool[])
    n180 = Boolean Array To Number(Boolean array=w274) -> (number=w273:u32)
    n181 = case shown="2" w273 {
      tunnel: w278 -> [w288 w313 w419 w601 w624]
      tunnel: w277 -> [w295 w312 w418 w600 _]
      tunnel: [w288 w325 w428 w605 w624] -> w272
      tunnel: [w295 w322 w427 w604 w623] -> w271
      tunnel: w262 -> [w292 w326 w444 _ w626]
      tunnel: "Save Volume" -> [_ w321 _ _ _]
      tunnel: w264 -> [_ _ w408 _ _]
      tunnel: w263 -> [_ _ w387 _ _]
      frame 0, Default {
        n182 = Unbundle(w292) -> ("queue out"=w291:refnum<queue>, "queue out"=w290:refnum<queue>, "queue out"=w289:refnum<queue>)
        n183 = call-dynamic "Read FPGA VI Reference.vi"("AODAcq in"=w288) -> ("FPGA VI Reference"=w279:T9)  [unwired: 8 in, 2 out]
        n184 = shared-variable "My Computer\\AODAcq.lvclass\\ReadFraction"(0.0 ("ReadFraction")) -> ()  [unwired: 1 in, 1 out]
        n185 = Wait (ms)(milliseconds to wait=u32 50) -> ()  [unwired: 1 out]
        n186 = Flush Queue(queue=w291) -> ()  [unwired: 1 in, 3 out]
        n187 = Flush Queue(queue=w290) -> ()  [unwired: 1 in, 3 out]
        n188 = Flush Queue(queue=w289) -> ()  [unwired: 1 in, 3 out]
        n189 = xnode "Invoke Method"("FPGA VI Reference In"=w279, "Number of Elements"=u32 0) -> ("Elements Remaining"=→"Motion samples remaining")  [unwired: 2 in, 3 out]
        n190 = xnode "Invoke Method"("FPGA VI Reference In"=w279, "Number of Elements"=u32 0) -> ("Elements Remaining"=→"Raw samples remaining")  [unwired: 2 in, 3 out]
        n191 = xnode "Invoke Method"("FPGA VI Reference In"=w279, "Number of Elements"=u32 0) -> ("Elements Remaining"=→"Temporal samples remaining")  [unwired: 2 in, 3 out]
        n192 = xnode "Invoke Method"("FPGA VI Reference In"=w279, "Number of Elements"=u32 0) -> ("Elements Remaining"=→"Image samples remaining")  [unwired: 2 in, 3 out]
        "Finished" <- FALSE ("Finished")
      }
      frame 1 {
        w305 = 2 ("dimension size")
        # "Volume imaging mode"
        n193 = local write "Volume"(FALSE ("Volume")) -> ()
        n194 = local write "Tab Control"(enum32{"Setup", "Volume", "Traces"}."Volume" ("Tab Control")) -> ()
        n195 = case shown="\"20x Olympus\", Default" "Objective" {
          tunnel: [T2 {"XStart"=1460000, "XEnd"=1460000, "XNum"=1, "YStart"=1460000, "YEnd"=1460000, "YNum"=1, "ZStart"=700, "ZEnd"=700, "ZNum"=1} ("y")] -> w341
          tunnel: [20] -> w298
          frame "20x Olympus", Default {
          }
        }
        "Lens Magnification" <- w298
        n196 = call-dynamic "Init.vi"("error in (no error)"=w312, "Channel"=i16 3, "AODAcq in"=w313) -> ("error out"=w311:errorcluster, "AODAcq out"=w310:refnum<class "AODAcq.lvclass">)  [unwired: 7 in]
        n197 = call "GetObjectivePosition.vi"() -> ("output cluster"=w299:cluster{"X":dbl, "Y":dbl, "Z":dbl})  [unwired: 8 in, 3 out]
        "Objective Position" <- w299
        n198 = call-dynamic "Reset.vi"("error in (no error)"=w311, "AODAcq in"=w310) -> ("error out"=w302:errorcluster, "AODAcq out"=w303:refnum<class "AODAcq.lvclass">)  [unwired: 8 in]
        n199 = Multiply(x=w341, y="Scan Settings (um)") -> (x*y=w344:T2)
        "Scan Settings" <- w344
        n200 = call-dynamic "Write Object Position.vi"("error in (no error)"=w302, "Object Position"=w299, "AODAcq in"=w303) -> ("error out"=w300:errorcluster, "AODAcq out"=w301:refnum<class "AODAcq.lvclass">)  [unwired: 7 in]
        n201 = Unbundle By Name("Scan Settings (um)") -> ("XNum"=w343:i32, "YNum"=w342:i32, "ZNum"=w307:i32)
        n202 = call-dynamic "Configure Volume.vi"("Save"=w321, "error in (no error)"=w300, "NumReps"="Volume Reps", "Scan Settings"=w344, "AODAcq in"=w301) -> ("error out"=w329:errorcluster, "AODAcq out"=w330:refnum<class "AODAcq.lvclass">)  [unwired: 5 in]
        n203 = call-dynamic "Start.vi"("error in (no error)"=w329, "AODAcq in"=w330) -> ("error out"=w317:errorcluster, "AODAcq out"=w319:refnum<class "AODAcq.lvclass">)  [unwired: 8 in]
        n204 = Select(t=w307, s="Disp Volume", f=u32 1) -> (s? t:f=w306:u32)
        n205 = call-dynamic "Read Recording File.vi"("error in (no error)"=w317, "AcquistionObject in"=w319) -> ("error out"=w316:errorcluster, "Recording File"=→"Recording File":path, "AcquistionObject out"=w318:refnum<class "AODAcq.lvclass">)  [unwired: 7 in]
        n206 = Compound Arithmetic op=MULTIPLY(w343, w342, w306) -> (w304:u32)
        n207 = call-dynamic "Read FPGA VI Reference.vi"("error in (no error)"=w316, "AODAcq in"=w318) -> ("error out"=w327:errorcluster, "FPGA VI Reference"=w333:T9, "AODAcq out"=w328:refnum<class "AODAcq.lvclass">)  [unwired: 7 in]
        n208 = Unbundle(w326) -> ("queue out"=w334:refnum<queue>, "queue out"=w331:refnum<queue>)  [unwired: 1 out]
        n209 = Initialize Array(0, w305, w304) -> (w340:i32[][])
        n210 = call-dynamic "Read Loop.vi"("error in (no error)"=w327, "ReadElements"="VolumeElements", "Queues"=w326, "AODAcq in"=w328) -> ("error out"=w323:errorcluster, "AODAcq out"=w324:refnum<class "AODAcq.lvclass">)  [unwired: 6 in]
        n211 = while {
          tunnel: w334 -> [w365]
          shift-right: [w361] -> _
          shift-left: w340 -> [w350]
          shift-right: [w362] -> _
          shift-left: 0 -> [w363]
          tunnel: w304 -> [w360]
          tunnel: 1000 ("timeout in ms (-1)") -> [w359]
          tunnel: w333 -> [w356]
          tunnel: w331 -> [w354]
          tunnel: w305 -> [w352]
          tunnel: w304 -> [w351]
          stop <- w357 stop-if-true
          n212 = Reshape Array(w350, w351, w352) -> ()  [unwired: 1 out]
          n213 = Flush Queue(queue=w354) -> ()  [unwired: 1 in, 3 out]
          n214 = local read "Abort"() -> (w353:bool)
          n215 = xnode "Read/Write Control"("FPGA VI Reference In"=w356, "Control.Abort"=w353) -> ()  [unwired: 1 in, 2 out]
          n216 = shared-variable "My Computer\\AODAcq.lvclass\\ReadFraction"() -> (→"Progress":dbl)  [unwired: 1 in, 1 out]
          n217 = Dequeue Element(queue=w365, timeout in ms (-1)=w359) -> (element=w364:waveform(i32)[], timed out?=w349:bool)  [unwired: 1 in, 2 out]
          n218 = shared-variable "My Computer\\AODAcq.lvclass\\ScanFraction"() -> (w355:dbl)  [unwired: 1 in, 1 out]
          n219 = case shown="True" w349 {
            tunnel: w350 -> [w371 w380]
            tunnel: w364 -> [w370 _]
            tunnel: w363 -> [w369 w379]
            tunnel: [w368 w379] -> w362
            tunnel: [w367 w380] -> w361
            tunnel: w360 -> [w366 _]
            tunnel: [_ w378] -> w357
            frame False {
              n220 = for {
                tunnel: w371 -> [w375] mode=indexing
                tunnel: w370 -> [w377] mode=indexing
                tunnel: [w376] -> w367 mode=indexing
                tunnel: w369 -> [w373]
                tunnel: [w374] -> w368
                tunnel: w366 -> [_]
                n221 = Unbundle By Name(w377) -> ("Y"=w372:i32[])
                n222 = call "WraparoundUpdate.vi"("Data"=w372, "Location"=w373, "Accumulator"=w375) -> ("NewLocation"=w374:u32, "Accumulated"=w376:i32[])  [unwired: 7 in]
              }
            }
            frame True {
              n223 = local read "Finished"() -> (w378:bool)
            }
          }
          "VolData" <- w361
          n224 = local write "ScanProgress"(w355) -> ()
        }
        n225 = flat-sequence {
          tunnel: w323 -> [_]
          tunnel: [FALSE] -> w320
          frame #0 {
            n226 = local write "Finished"(TRUE ("Finished")) -> ()
          }
        }
        n227 = call-dynamic "Stop.vi"("error in (no error)"=w323, "AODAcq in"=w324) -> ("error out"=w322:errorcluster, "AODAcq out"=w325:refnum<class "AODAcq.lvclass">)  [unwired: 8 in]
        n228 = local write "Save Volume"(w320) -> ()
      }
      frame 2 {
        (unwired) 0
        # "Point imaging mode"
        n229 = Flush Queue(queue=w387) -> (queue out=w386:refnum<queue>)  [unwired: 1 in, 2 out]
        n230 = global write "GlobalVars.vi" "Scanning"(TRUE ("Scanning")) -> ()
        n231 = local write "Scan"(FALSE ("Scan")) -> ()
        n232 = call-dynamic "Init.vi"("error in (no error)"=w418, "Channel"=i16 3, "AODAcq in"=w419) -> ("error out"=w413:errorcluster, "AODAcq out"=w410:refnum<class "AODAcq.lvclass">)  [unwired: 7 in]
        n233 = call "GetObjectivePosition.vi"() -> ("output cluster"=w409:cluster{"X":dbl, "Y":dbl, "Z":dbl})  [unwired: 8 in, 3 out]
        n234 = local read "Scan Settings (um)"() -> (w394:T2)
        n235 = local read "Number selected"() -> (w400:u32)
        n236 = local write "Tab Control"(enum32{"Setup", "Volume", "Traces"}."Traces" ("Tab Control")) -> ()
        n237 = local write "Objective Position"(w409) -> ()
        n238 = call-dynamic "Write Object Position.vi"("error in (no error)"=w413, "Object Position"=w409, "AODAcq in"=w410) -> ("error out"=w412:errorcluster, "AODAcq out"=w411:refnum<class "AODAcq.lvclass">)  [unwired: 7 in]
        n239 = local read "Scan Settings"() -> (w395:T2)
        n240 = call-dynamic "Reset.vi"("error in (no error)"=w412, "AODAcq in"=w411) -> ("error out"=w453:errorcluster, "AODAcq out"=w406:refnum<class "AODAcq.lvclass">)  [unwired: 8 in]
        n241 = local read "Motion Points (Ch1)"() -> (w393:u32)
        n242 = local read "Motion rate (Hz)"() -> (w396:dbl)
        n243 = local read "Motion ROIs"() -> (w399:T1)
        n244 = local read "GridPoints"() -> (w397:u16)
        n245 = call-dynamic "ConfigurePerCellMotionAnalysis.vi"("Scan Settings (um)"=w394, "Points Selected"=w400, "Scan Settings"=w395, "Sampling Structure"="Sampling Structure", "Per Cell Motion Analysis"="Per Cell Motion Analysis", "In Points"="Points", "AODAcq in"=w406) -> ("Additional Points"=w403:i32, "Out Points"=w398:i32[][])  [unwired: 1 in, 2 out]
        n246 = case shown="True" "Per Cell Motion Analysis" {
          tunnel: w400 -> [w455 w459]
          tunnel: w403 -> [_ w458]
          tunnel: [w455 w456] -> w402
          frame False {
          }
          frame True {
            n247 = Multiply(x=w459, y=w458) -> (x*y=w457:u32)
            n248 = Add(x=w459, y=w457) -> (x+y=w456:u32)
          }
        }
        n249 = call "AutoConfigureAdditionalMotionPlanes.vi"("Motion ROIs"=w399, "Number of Motion Points"=w393, "Plane Params"="Auto Motion Plane Params", "In Points"=w398, "Grid Points"=w397, "Motion Rate (Hz)"=w396, "Scan Settings"=w395, "Scan Settings (um)"=w394) -> ("X-Y Motion Points"=w389:i32[][], "Out Points"=w391:i32[][], "Total Motion Points"=w392:i32, "Motion Increment"=w390:i32, "Y-Z Motion Points"=w388:i32[][])  [unwired: 1 in, 2 out]
        "Out Points" <- w391
        "Total Motion Points" <- w392
        n250 = local read "GridPoints"() -> (w437:u16)
        n251 = Initialize Array(0 ("element"), w392) -> ()  [unwired: 1 out]
        n252 = Quotient & Remainder(x=w392, y=w437) -> (floor(x/y)=w438:i32)  [unwired: 1 out]
        n253 = local write "X-Y Motion Points"(w389) -> ()
        n254 = local write "Motion Increment"(w390) -> ()
        n255 = local write "Y-Z Motion Points"(w388) -> ()
        n256 = Multiply(x="Scan Time (s)", y=50000.0) -> (x*y=w450:dbl)
        n257 = Decrement(x=w390) -> (x-1=w431:i32)
        n258 = Divide(x=w450, y=w402) -> (x/y=w433:dbl)
        n259 = Divide(x=w431, y=w390) -> (x/y=w430:dbl)
        n260 = Quotient & Remainder(x="TraceElements", y=w402) -> (floor(x/y)=w446:u32)  [unwired: 1 out]
        n261 = disable-structure shown="Disabled" {
          disable-tunnel: [w454 _] -> w383
          frame Disabled {
            n262 = script code="load z:\\users\\spatel\\temp\\ch1lindata"() -> ("ch1lindata"=w454:dbl[][])  [unwired: 1 in, 1 out]
          }
          frame Enabled {
          }
        }
        n263 = Multiply(x=w402, y=w446) -> (x*y=w445:u32)
        n264 = Multiply(x=w430, y=w433) -> (x*y=w432:dbl)
        n265 = call-dynamic "Configure PointScan.vi"("AODAcq in"=w406, "Save"=TRUE ("Save Volume"), "Store Raw"="Store Raw", "Points"=w391, "GridSize"=w397, "Reps"=w432, "error in (no error)"=w453, "Motion Points"=w392, "Motion Increment"=w390) -> ("AODAcq out"=w441:refnum<class "AODAcq.lvclass">, "error out"=w442:errorcluster)  [unwired: 5 in]
        n266 = Unbundle(w444) -> ("queue out"=w443:refnum<queue>, "queue out"=w439:refnum<queue>)  [unwired: 1 out]
        n267 = call-dynamic "Read FPGA VI Reference.vi"("error in (no error)"=w442, "AODAcq in"=w441) -> ("error out"=w426:errorcluster, "FPGA VI Reference"=w440:T9, "AODAcq out"=w425:refnum<class "AODAcq.lvclass">)  [unwired: 7 in]
        n268 = call-dynamic "Start.vi"("error in (no error)"=w426, "AODAcq in"=w425) -> ("error out"=w422:errorcluster, "AODAcq out"=w424:refnum<class "AODAcq.lvclass">)  [unwired: 8 in]
        n269 = while {
          tunnel: w402 -> [w499]
          tunnel: 300 ("timeout in ms (-1)") -> [w489]
          tunnel: w446 -> [w494]
          tunnel: w443 -> [w492]
          tunnel: w440 -> [w491]
          tunnel: w439 -> [w485]
          tunnel: w438 -> [_]
          tunnel: w437 -> [w472]
          border: 0 -> [_]
          tunnel: w408 -> [w481]
          tunnel: w392 -> [w467]
          tunnel: w386 -> [w469]
          shift-right: [w461] -> _
          shift-left: 0 -> [w462]
          tunnel: w383 -> [w465]
          i -> [w484]
          stop <- w478 stop-if-true
          n270 = disable-structure shown="Disabled" {
            disable-tunnel: w465 -> [w509 _]
            disable-tunnel: w462 -> [w508 _]
            frame Disabled {
              w505 = 1200 ("length")
              n271 = Multiply(x=w508, y=w505) -> (x*y=w507:i32)
              n272 = Array Subset(array=w509, index (row)=w507, length (row)=w505) -> (w506:dbl[][])  [unwired: 2 in]
              n273 = Reshape Array(w506, w505) -> (w504:dbl[])
              n274 = To Long Integer(number=w504) -> ()  [unwired: 1 out]
            }
            frame Enabled {
            }
          }
          n275 = Dequeue Element(queue=w492, timeout in ms (-1)=w489) -> (element=w503:waveform(i32)[])  [unwired: 1 in, 3 out]
          n276 = Dequeue Element(queue=w485, timeout in ms (-1)=w489) -> (element=w480:waveform(i32)[])  [unwired: 1 in, 3 out]
          n277 = Square(x=w472) -> (x^2=w466:u16)
          n278 = local read "Finished"() -> (w482:bool)
          n279 = Divide(x=50000, y=w499) -> (x/y=w498:dbl)
          n280 = shared-variable "My Computer\\AODAcq.lvclass\\ReadFraction"() -> (w487:dbl)  [unwired: 1 in, 1 out]
          n281 = shared-variable "My Computer\\AODAcq.lvclass\\ScanFraction"() -> (→"ScanProgress":dbl)  [unwired: 1 in, 1 out]
          n282 = xnode "Read/Write Control"("FPGA VI Reference In"=w491, "Control.Abort"="Abort") -> ()  [unwired: 1 in, 2 out]
          n283 = Divide(x=w467, y=w466) -> (x/y=w475:dbl)
          n284 = Divide(x=w498, y="Down Rate") -> (x/y=w501:dbl)
          n285 = Divide(x=w475, y=2.0) -> (x/y=w473:dbl)
          n286 = Not Equal To 0?(x=w484) -> (x != 0?=w483:bool)
          n287 = Round To Nearest(number=w501) -> (nearest integer value=w496:dbl)
          n288 = Increment(x=w473) -> (x+1=w471:dbl)
          n289 = And(x=w482, y=w483) -> (x .and. y?=w478:bool)
          n290 = local write "Progress"(w487) -> ()
          n291 = Multiply(x=w471, y=w466) -> (x*y=w470:dbl)
          n292 = Decrement(x="Motion Channel To Analyze") -> (x-1=w476:i32)
          n293 = In Range and Coerce(upper limit=w494, x=w496, lower limit=1.0) -> (coerced(x)=w493:dbl)  [unwired: 1 out]
          n294 = Not(x=w478) -> (.not. x?=w479:bool)
          n295 = case shown="\"Traces\"" "Tab Control" {
            tunnel: w499 -> [_ w578]
            tunnel: w503 -> [_ w584]
            tunnel: w493 -> [_ w581]
            frame Default {
            }
            frame "Traces" {
              n296 = Index Array(array=w584, index=0) -> (element=w565:waveform(i32))
              n297 = Add(x=w565, y="Baseline Offset") -> (x+y=w563:waveform(dbl))
              n298 = Unbundle By Name(w563) -> ("dt"=w586:dbl, "Y"=w583:dbl[])
              n299 = Multiply(x=w578, y=w586) -> (x*y=w585:dbl)
              n300 = Array Size(array=w583) -> (size(s)=w573:i32)
              n301 = Divide(x=w573, y=w578) -> (x/y=w577:dbl)
              n302 = feedback #1() -> (w572:i32)
              n303 = Add(x=w573, y=w572) -> (x+y=w568:i32)
              n304 = feedback-in #1(w568) -> ()
              n305 = Reshape Array(w583, w577, w578) -> (w576:dbl[][])
              n306 = Less?(x=w568, y=50000) -> (x < y?=w566:bool)
              n307 = Transpose 2D Array(2D array=w576) -> (transposed array=w575:dbl[][])
              n308 = for {
                tunnel: w585 -> [w597]
                tunnel: w563 -> [w596]
                tunnel: [w595] -> w580 mode=indexing
                tunnel: w575 -> [w594] mode=indexing
                n309 = Bundle By Name(cluster=w596, "dt"=w597, "Y"=w594) -> (w595:waveform(dbl))
              }
              n310 = Select(t=1.0, s=w566, f=0.001 ("Baseline Rate")) -> (s? t:f=w569:dbl)
              n311 = case shown="True" "Decimate" {
                tunnel: "Spacing" -> [_ w593]
                tunnel: w581 -> [_ w592]
                tunnel: w580 -> [w588 w591]
                tunnel: [w588 w590] -> w579
                tunnel: w569 -> [_ w589]
                frame False {
                }
                frame True {
                  n312 = call "CleanupTraces.vi"("Baseline Rate"=w589, "Spacing"=w593, "decimating factor"=w592, "Traces in"=w591) -> ("Traces out"=w590:waveform(dbl)[])  [unwired: 7 in]
                }
              }
              "Traces" <- w579
            }
          }
          n313 = Index Array(array=w480, index=w476) -> (element=w488:waveform(i32))
          n314 = global write "GlobalVars.vi" "Scanning"(w479) -> ()
          n315 = Unbundle By Name(w488) -> ("Y"=w463:i32[])
          n316 = call "Motion FIFO.vi"("Packet Length"=w467, "Data"=w463, "Motion FIFO"=w469) -> ("Number of Packets"=w468:i32, "Array"=w464:i32[])  [unwired: 7 in]
          n317 = for {
            N: w468 -> [_]
            tunnel: w481 -> [w529]
            tunnel: w472 -> [w517]
            tunnel: w470 -> [w527]
            tunnel: w464 -> [w526]
            tunnel: w467 -> [w520]
            tunnel: w466 -> [w519]
            tunnel: w462 -> [w513]
            tunnel: w462 -> [w511]
            tunnel: [w510] -> w461
            i -> [w512]
            n318 = Multiply(x=w520, y=w512) -> (x*y=w525:i32)
            n319 = Array Subset(array=w526, index=w525, length=w520) -> (w515:i32[])
            n320 = Array Size(array=w515) -> (size(s)=w514:i32)
            n321 = Array Subset(array=w515, index=w527, length=w519) -> (w522:i32[])
            n322 = Array Subset(array=w515, index=w519, length=w519) -> (w521:i32[])
            n323 = Reshape Array(w522, w517, w517) -> (w528:i32[][])
            n324 = Reshape Array(w521, w517, w517) -> (w524:i32[][])
            n325 = Insert Into Array(array=w524, new element=w528) -> (w523:i32[][])  [unwired: 2 in]
            n326 = Reshape Array(w515, 1 ("dimension size"), w514) -> (w518:i32[][])
            n327 = local read "Motion Ch1"() -> (w532:T4)
            n328 = case shown="True" "Motion Analysis" {
              tunnel: w529 -> [_ w556]
              tunnel: w518 -> [_ w550]
              tunnel: w517 -> [_ w551]
              tunnel: w513 -> [_ w545]
              tunnel: w512 -> [_ w544]
              tunnel: w511 -> [w534 w540]
              tunnel: [w534 w539] -> w510
              frame False {
                n329 = global read "GlobalVars.vi" "VI Open"() -> (w535:bool)
                n330 = case shown="True" w535 {
                  frame False {
                  }
                  frame True {
                    n331 = global write "GlobalVars.vi" "VI Open"(FALSE ("VI Open")) -> ()
                    n332 = vi-ref "RunDuringExperiment.vi"() -> (w537:refnum<vi>)
                    n333 = invoke on="Invoke Node" class="VI" method="Abort VI"(reference=w537) -> (reference out=w538:refnum<vi>)  [unwired: 2 in, 2 out]
                    n334 = invoke class="VI" method="FP.Close"(reference=w538) -> ()  [unwired: 2 in, 3 out]
                  }
                }
              }
              frame True {
                n335 = Equal To 0?(x=w544) -> (x = 0?=w543:bool)
                n336 = Equal To 0?(x=w545) -> (x = 0?=w542:bool)
                n337 = global read "GlobalVars.vi" "VI Open"() -> (w555:bool)
                n338 = local read "Scan Settings (um)"() -> (w553:T2)
                n339 = local read "X-Y Motion Points"() -> (w558:i32[][])
                n340 = local read "Y-Z Motion Points"() -> (w557:i32[][])
                n341 = local read "Scan Settings"() -> (w554:T2)
                n342 = case shown="False" w555 {
                  frame False {
                    n343 = vi-ref "RunDuringExperiment.vi"() -> (w562:refnum<vi>)
                    n344 = invoke on="Invoke Node" class="VI" method="FP.Open"(reference=w562) -> (reference out=w561:refnum<vi>)  [unwired: 4 in, 4 out]
                    n345 = invoke class="VI" method="Run VI"(reference=w561, "Wait until done"=FALSE ("Wait Until Done"), "Auto Dispose Ref"=TRUE ("Auto Dispose Reference")) -> ()  [unwired: 2 in, 5 out]
                  }
                  frame True {
                  }
                }
                n346 = And(x=w543, y=w542) -> (x .and. y?=w541:bool)
                n347 = Cluster To Array(cluster=w554) -> (array=w548:i32[])
                n348 = Cluster To Array(cluster=w553) -> (array=w547:i32[])
                n349 = Insert Into Array(array=w558, new element=w557) -> (w549:i32[][])  [unwired: 2 in]
                n350 = Bundle By Name(cluster=T5 {"gridsize"=0, "data"=[], "coordinates"=[], "settings"=[], "settings_um"=[], "needsreference"=FALSE}, "gridsize"=w551, "data"=w550, "coordinates"=w549, "settings"=w548, "settings_um"=w547, "needsreference"=w541) -> (w546:T5)
                n351 = Increment "Loop Counter"(x=w540) -> (x+1=w539:i32)
                n352 = Lossy Enqueue Element(queue=w556, element=w546) -> ()  [unwired: 1 in, 4 out]
              }
            }
            n353 = To Single Precision Float(number=w523) -> (single precision float=w531:sgl[][])
            n354 = call "IMAQ ArrayToImage"("Image Pixels (Float)"=w531, "Image"=w532) -> ("Image Out"=w533:T4)  [unwired: 8 in, 1 out]
            n355 = local write "Motion Ch1"(w533) -> ()
          }
        }
        n356 = call-dynamic "Read Recording File.vi"("error in (no error)"=w422, "AcquistionObject in"=w424) -> ("error out"=w416:errorcluster, "Recording File"=w421:path, "AcquistionObject out"=w423:refnum<class "AODAcq.lvclass">)  [unwired: 7 in]
        n357 = local write "Recording File"(w421) -> ()
        n358 = call-dynamic "Read Loop.vi"("error in (no error)"=w416, "ReadElements"=w445, "Queues"=w444, "AODAcq in"=w423) -> ("error out"=w415:errorcluster, "AODAcq out"=w429:refnum<class "AODAcq.lvclass">)  [unwired: 6 in]
        n359 = flat-sequence {
          tunnel: w415 -> [_]
          frame #0 {
            n360 = local write "Finished"(TRUE ("Finished")) -> ()
          }
        }
        n361 = call-dynamic "Stop.vi"("error in (no error)"=w415, "AODAcq in"=w429) -> ("error out"=w427:errorcluster, "AODAcq out"=w428:refnum<class "AODAcq.lvclass">)  [unwired: 8 in]
      }
      frame 4 {
        n362 = call-dynamic "Reset.vi"("error in (no error)"=w600, "AODAcq in"=w601) -> ("error out"=w599:errorcluster, "AODAcq out"=w598:refnum<class "AODAcq.lvclass">)  [unwired: 8 in]
        n363 = call-dynamic "Read FPGA VI Reference.vi"("error in (no error)"=w599, "AODAcq in"=w598) -> ("error out"=w607:errorcluster, "FPGA VI Reference"=w608:T9, "AODAcq out"=w606:refnum<class "AODAcq.lvclass">)  [unwired: 7 in]
        n364 = flat-sequence {
          tunnel: w608 -> [w611]
          tunnel: w607 -> [w609]
          tunnel: w606 -> [w610]
          tunnel: [w610] -> w603
          tunnel: [w609] -> w602
          tunnel: [w613] -> w604
          tunnel: [w612] -> w605
          tunnel: w603 -> [w615]
          tunnel: w602 -> [w614]
          frame #0 {
            n365 = call "SweepSettings.vi"("FPGA VI Reference Out"=w611) -> ()  [unwired: 11 in]
          }
          frame #1 {
            n366 = call-dynamic "GetStatus.vi"("error in (no error)"=w614, "AODAcq in"=w615) -> ("error out"=w613:errorcluster, "AODAcq out"=w612:refnum<class "AODAcq.lvclass">)  [unwired: 7 in, 1 out]
          }
        }
      }
      frame 8 {
        n367 = Unbundle(w626) -> ("queue out"=w620:refnum<queue>)  [unwired: 2 out]
        n368 = local write "Ephys"(FALSE ("Ephys")) -> ()
        n369 = local write "Ephys"(TRUE ("Ephys")) -> ()
        n370 = local write "Tab Control"(enum32{"Setup", "Volume", "Traces", "Motion"}."Traces" ("Tab Control")) -> ()
        n371 = call "DAQ Assistant"() -> ("task out"=w627:refnum<k21>, "error out"=w622:errorcluster)  [unwired: 16 in, 2 out]
        n372 = while {
          tunnel: w627 -> [w636]
          tunnel: w620 -> [w635]
          tunnel: [w634] -> w625
          tunnel: w622 -> [w633]
          tunnel: [w631] -> w621
          tunnel: [FALSE ("Ephys")] -> w617
          stop <- w637 stop-if-true
          n373 = call-poly <vilib>:"DAQmx Read.vi"("task/channels in"=w636, "error in"=w633) -> ("task out"=w634:refnum<k21>, "data"=w629:waveform(dbl), "error out"=w632:errorcluster)  [unwired: 11 in]
          "Waveform Chart" <- w629
          n374 = Build Array(w629) -> (w628:waveform(dbl)[])
          n375 = Enqueue Element(queue=w635, element=w628, error in (no error)=w632) -> (error out=w631:errorcluster)  [unwired: 1 in, 2 out]
          n376 = local read "Abort"() -> (w637:bool)
        }
        "Ephys" <- w617
        n377 = call <vilib>:"DAQmx Clear Task.vi"("task in"=w625, "error in"=w621) -> ("error out"=w623:errorcluster)  [unwired: 13 in]
      }
    }
    "AODAcq out" <- w272
    n378 = call <vilib>:"Simple Error Handler.vi"("error in (no error)"=w271) -> ("error out"=w270:errorcluster)  [unwired: 4 in, 4 out]
    "Volume" <- "Volume"
    "Scan" <- "Scan"
    "Numeric" <- w265
  }
  "Stopped" <- w12
  n379 = while {
    tunnel: w26 -> [w640]
    stop <- w639 stop-if-true
    n380 = local read "Tab Control"() -> (w638:enum32{"Setup", "Volume", "Traces", "Motion"})
    n381 = case shown="\"Traces\"" w638 {
      tunnel: w640 -> [_ w646]
      frame "Setup", Default {
        n382 = Wait (ms)(milliseconds to wait=u32 150) -> ()  [unwired: 1 out]
      }
      frame "Traces" {
        n383 = Dequeue Element(queue=w646, timeout in ms (-1)=500) -> (element=w643:waveform(dbl)[], timed out?=w642:bool, error out=w644:errorcluster)  [unwired: 1 in, 1 out]
        n384 = call <vilib>:"Clear Errors.vi"("error in (no error)"=w644) -> ()  [unwired: 6 in, 1 out]
        n385 = case shown="False" w642 {
          tunnel: w643 -> [w647 _]
          frame False {
            "Ephys" <- w647
          }
          frame True {
          }
        }
      }
    }
    n386 = local read "Stopped"() -> (w639:bool)
  }
  n387 = case shown="True" w12 {
    tunnel: [errorcluster {"status"=FALSE, "code"=0, "source"=""} ("error out") w650] -> w13
    frame False {
    }
    frame True {
      n388 = global read "GlobalVars.vi" "VI Open"() -> (w649:bool)
      n389 = case shown="True" w649 {
        tunnel: [errorcluster {"status"=FALSE, "code"=0, "source"=""} ("error out") w654] -> w650
        frame False {
        }
        frame True {
          n390 = vi-ref "RunDuringExperiment.vi"() -> (w652:refnum<vi>)
          n391 = invoke on="Invoke Node" class="VI" method="Abort VI"(reference=w652) -> (reference out=w653:refnum<vi>)  [unwired: 2 in, 2 out]
          n392 = invoke class="VI" method="FP.Close"(reference=w653) -> (error out=w654:errorcluster)  [unwired: 2 in, 2 out]
        }
      }
    }
  }
  n393 = stacked-sequence {
    tunnel: w13 -> [_ w658]
    frame #0 {
      n394 = Wait Until Next ms Multiple(millisecond multiple=u32 100) -> ()  [unwired: 1 out]
    }
    frame #1 {
      n395 = local read "Motion FIFO"() -> (w657:refnum<queue>)
      n396 = global read "GlobalVars.vi" "MotionAnalysis"() -> (w656:refnum<queue>)
      n397 = Release Queue(queue=w657) -> ()  [unwired: 2 in, 3 out]
      n398 = Release Queue(queue=w656, error in (no error)=w658) -> ()  [unwired: 1 in, 3 out]
    }
  }
  "Points_um" <- dbl[][] [] ("Points_um")
